vi "SwissSPAD Live_Write HDF5 Header.vi"(8 "error in (no error)":errorcluster, 9 "Gate Names":string[](array[string]), 10 "Current Data Set":i32, 11 "ref in":T1 format="%.0x") -> (0 "Error Out":errorcluster, 1 "Notebook Message":string, 2 "# Image Sets":u32, 3 "ref out":T1 format="%.0x", 5 "# Datasets in Series":i32)   [LabVIEW 2021]
uses:
  <vilib>/addons/h5labview2/base/hid_t.ctl
  SwissSPAD Live_HDF5 Header Sections.ctl
  SwissSPAD Live_File Information.ctl
  SwissSPAD Live_Settings List.ctl
  SwissSPAD Live_SSx PCB Version.ctl
  SwissSPAD Live_Image ROI Information.ctl
  Phasor/Image Binning Options.ctl
  <vilib>/addons/h5labview2/base/lib_path.vi
  <vilib>/addons/h5labview2/base/H5Equery.vi
  <vilib>/addons/h5labview2/dataset/H5Dwrite.llb/H5Dwrite.xnode
  <vilib>/addons/h5labview2/group/H5G.lvlib
  Variant/Variant to Data/Variant to Data.lvlib
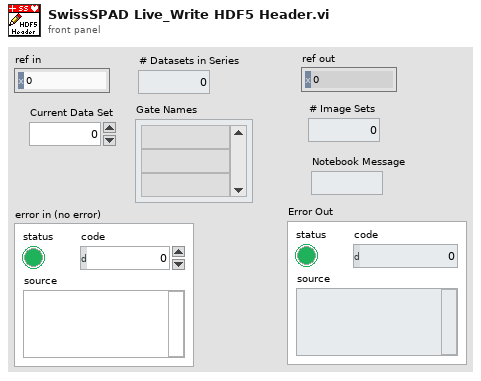
[diagram p1: front panel]
types:
  T1 = typedef "hid_t.ctl" = i32
  T2 = typedef "SwissSPAD Live_HDF5 Header Sections.ctl" = enum16{"File Information", "SwissSPAD Detector Information", "DAQ Parameters", "Image Information", "Metadata"}
  T3 = typedef "SwissSPAD Live_Settings List.ctl" = enum16{"FPGA:Bottom Half", "FPGA:Top Half", "FPGA:Bottom Bitfile Path", "FPGA:Top Bitfile Path", "FPGA:Bottom Bitstream Version", "FPGA:Top Bitstream Version", "FPGA:Auto Reset FPGA", "FPGA:Bottom FPGA Serial Number", "FPGA:Top FPGA Serial Number", "FPGA:Detector PCB Version", "Acquisition Parameters:Microlens", "Acquisition Parameters:SS2 DAQ Parameters", "Acquisition Parameters:Gate Configuration Array", "Acquisition Parameters:SS3 DAQ Parameters", "Acquisition Parameters:Buffer Size (# 8-bit Gates)", "File Information:File Information", "File Information:# Datasets in Series", "File Information:Scrambled File Flag", "File Information:SS3 Gate Slip Correction", "File Information:SS3 Hot Pixel Mismatch Detection", "File Information:Delay between Datasets", "File Information:Save Sum of All Gates Preview", "Image Parameters:Image ROI Information", "Image Parameters:Image Binning Options", "Image Parameters:SS3 Displayed Image", "Image Parameters:Image Display Options", "Image Parameters:Use Histogram Cursors", "Image Parameter:FPGA Data to Display", "UI Settings:Histogram Bins Number", "UI Settings:Use Image Display Options", "UI Settings:Verbose Settings", "UI Settings:Verbose Saving"}
  T4 = typedef "SwissSPAD Live_File Information.ctl" = cluster{"File Folder":path, "File Name":string, "File Index":u32, "Author":string, "Sample":string, "Compression":bool, "Compression Level":u8}
  T5 = typedef "SwissSPAD Live_SSx PCB Version.ctl" = enum16{"unknown", "SS2 PCB1", "SS2 PCB2", "SS3 PCB1"}
  T6 = typedef "Image Binning Options.ctl" = cluster{"Use Image Binning":bool, "X Bin":i32, "Y Bin":i32}
  T7 = typedef "SwissSPAD Live_Image ROI Information.ctl" = cluster{"Save ROI Only":bool, "Left":u16, "Top":u16, "Right":u16, "Bottom":u16, "Use Current ROI":bool}
  T8 = typedef "Fluorescence Lifetime Parameters v3.ctl" = cluster{"# Pixel X":i32, "# Pixel Y":i32, "# Gates":i32, "# Datasets":i32, "Gate Image Exposure":dbl[unit], "Macrotime Gate Separation":dbl[unit], "Nanotime Gate Separation":dbl[unit], "Gate Width":dbl[unit], "Laser Period":dbl[unit], "SYNC Period":dbl[unit], "Gate Image Integration":dbl[unit]}
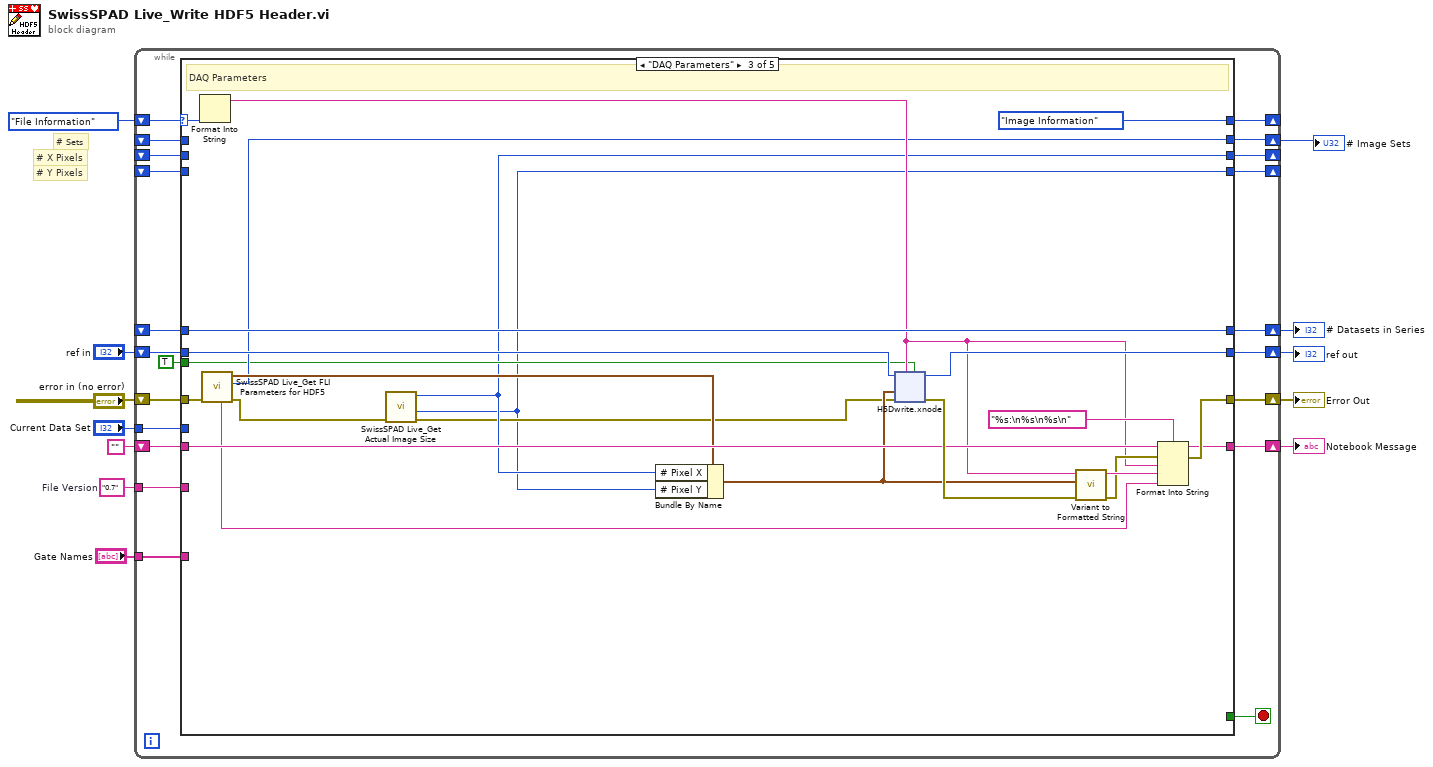
[diagram p0: block diagram]
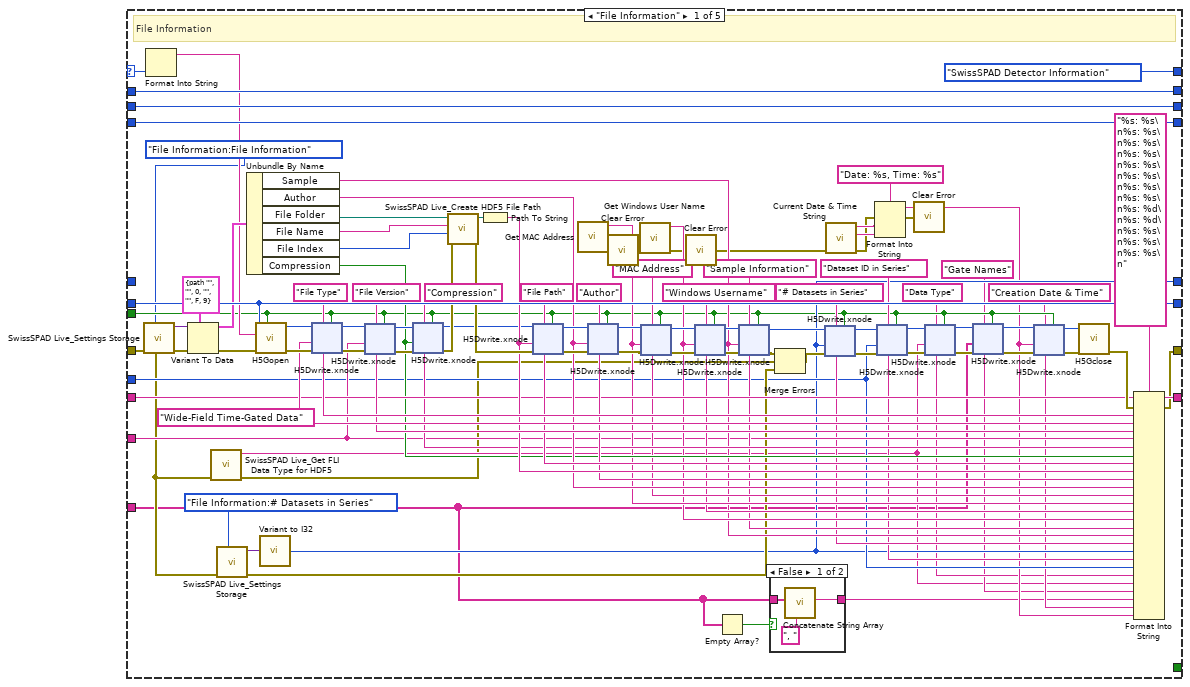
[diagram p2: hidden frame]
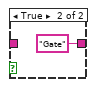
[diagram p3: hidden frame]
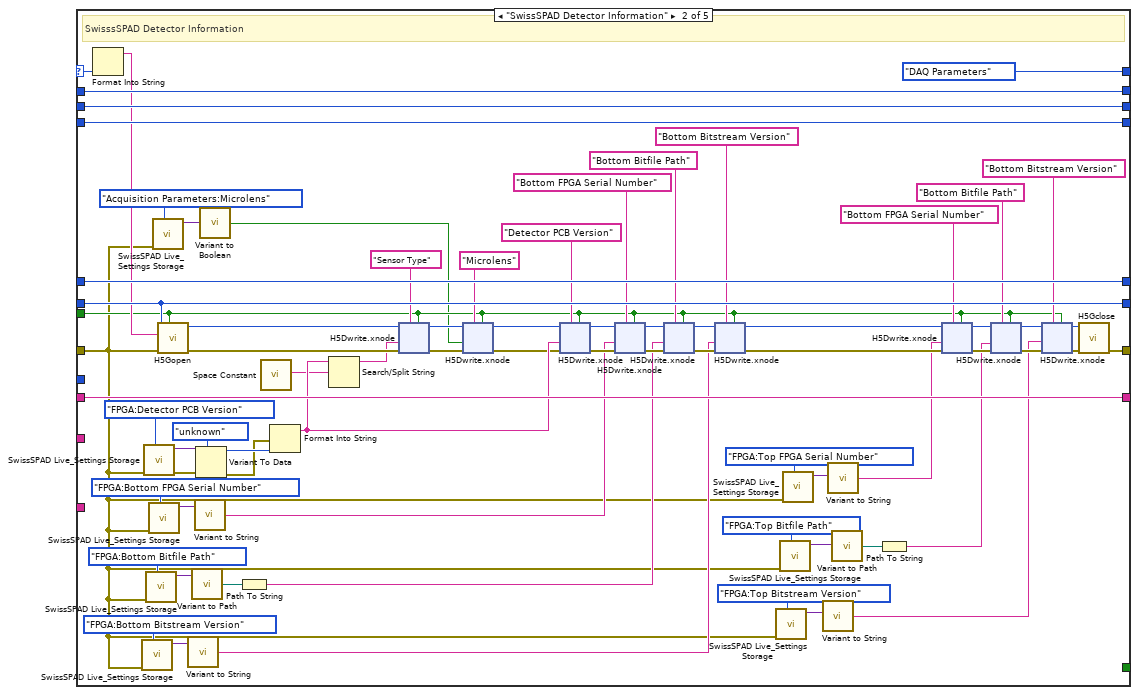
[diagram p4: hidden frame]
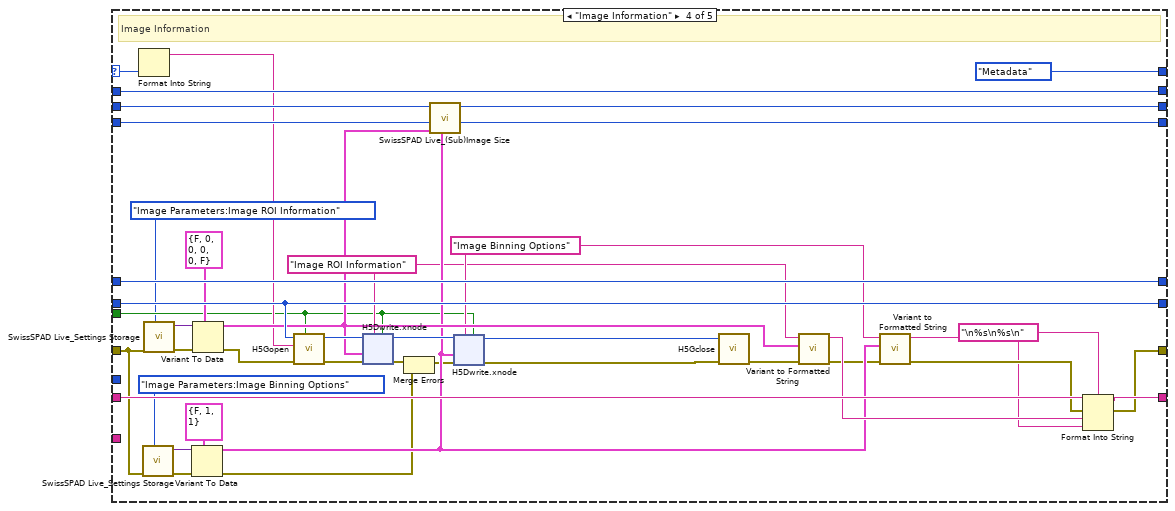
[diagram p5: hidden frame]
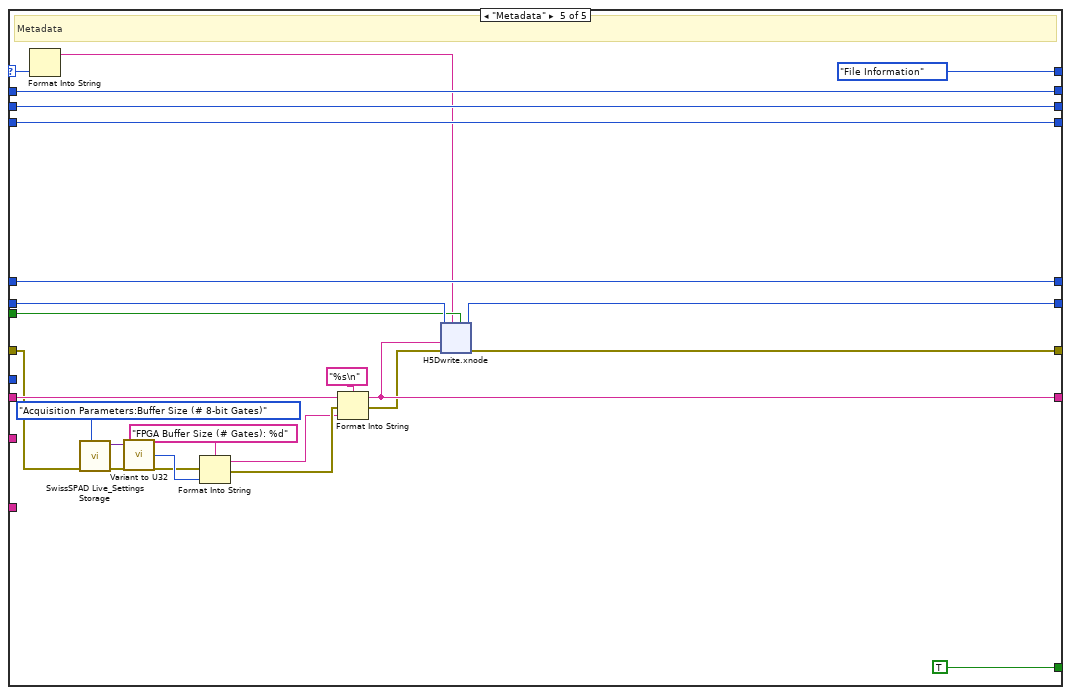
[diagram p6: hidden frame]
diagram:
  w3 = "0.7"  # File Version
  # "# Y Pixels"
  # "# X Pixels"
  # "# Sets"
  n1 = while {
    shift-right: [w30] -> w10
    shift-left: "ref in" -> [w32]
    shift-right: [w31] -> w9
    shift-left: "error in (no error)" -> [w33]
    shift-right: [w27] -> w6
    shift-left: _ -> [w26]
    tunnel: "Current Data Set" -> [w25]
    shift-right: [w24] -> w7
    shift-left: _ -> [w23]
    shift-right: [w28] -> w4
    shift-left: "" -> [w22]
    shift-right: [w20] -> _
    shift-left: _ -> [w21]
    shift-right: [w18] -> _
    shift-left: _ -> [w19]
    tunnel: w3 -> [w17]
    shift-right: [w15] -> _
    shift-left: SwissSPAD_Live_HDF5_Header_Sections."File Information" -> [w16]
    tunnel: "Gate Names" -> [w13]
    stop <- w14 stop-if-true
    n2 = case shown="\"DAQ Parameters\"" w16 {
      selector: w16 -> [w72 w445 w630 w679 w750]
      tunnel: w33 -> [w54 w383 w645 w687 w756]
      tunnel: w32 -> [w122 w446 w639 w705 w768]
      tunnel: [w96 w442 w641 w697 w759] -> w31
      tunnel: [w122 w446 w644 w705 w767] -> w30
      tunnel: TRUE ("replace? (F)") -> [w47 w384 w627 w672 w766]
      tunnel: [w99 w441 w638 w698 w761] -> w28
      tunnel: [w55 w451 w636 w701 w764] -> w27
      tunnel: w26 -> [_ w451 w636 w701 w764]
      tunnel: w25 -> [w61 _ _ _ _]
      tunnel: [w95 w450 w628 w702 w763] -> w24
      tunnel: w23 -> [w95 w450 _ w702 w763]
      tunnel: w22 -> [w94 w441 w637 w699 w762]
      tunnel: [w93 w449 w626 w693 w758] -> w20
      tunnel: w21 -> [w93 w449 _ w694 w758]
      tunnel: [w92 w448 w623 w691 w757] -> w18
      tunnel: w19 -> [w92 w448 _ w692 w757]
      tunnel: w17 -> [w73 _ _ _ _]
      tunnel: [SwissSPAD_Live_HDF5_Header_Sections."SwissSPAD Detector Information" SwissSPAD_Live_HDF5_Header_Sections."DAQ Parameters" SwissSPAD_Live_HDF5_Header_Sections."Image Information" SwissSPAD_Live_HDF5_Header_Sections."Metadata" SwissSPAD_Live_HDF5_Header_Sections."File Information"] -> w15
      tunnel: [_ _ _ _ TRUE] -> w14
      tunnel: w13 -> [w39 _ _ _ _]
      frame "File Information" {
        w43 = "Gate Names" ("dataset name")
        w44 = "Data Type" ("dataset name")
        w62 = "Dataset ID in Series" ("name")
        w63 = "# Datasets in Series" ("name")
        w77 = "Windows Username" ("dataset name")
        w79 = "MAC Address" ("dataset name")
        w87 = "Compression" ("dataset name")
        w45 = "Creation Date & Time" ("dataset name")
        w75 = "Sample Information" ("dataset name")
        w101 = "Author" ("dataset name")
        w103 = "File Path" ("dataset name")
        w105 = "Wide-Field Time-Gated Data" ("dataset name")
        w106 = "File Type" ("dataset name")
        w104 = "File Version" ("dataset name")
        # "File Information"
        n3 = call "SwissSPAD Live_Settings Storage.vi"("Settings List"=SwissSPAD_Live_Settings_List."File Information:File Information", "Error In"=w54) -> ("Error Out"=w128:errorcluster, "Variant Data out"=w36:variant)  [unwired: 8 in]
        n4 = Format Into String(w72) -> (resulting string=w71:string)  [unwired: 3 in, 1 out]
        n5 = Variant To Data(error in=w128, type=T4 {"File Folder"=path "", "File Name"="", "File Index"=0, "Author"="", "Sample"="", "Compression"=FALSE, "Compression Level"=9} ("File Information"), Variant=w36) -> (data=w120:T4, error out=w121:errorcluster)
        n6 = call "SwissSPAD Live_Get FLI Data Type for HDF5.vi"("error in (no error)"=w54) -> ("error out"=w41:errorcluster, "Data Type"=w42:string)  [unwired: 9 in]
        n7 = call "SwissSPAD Live_Settings Storage.vi"("Settings List"=SwissSPAD_Live_Settings_List."File Information:# Datasets in Series", "Error In"=w54) -> ("Error Out"=w64:errorcluster, "Variant Data out"=w34:variant)  [unwired: 8 in]
        n8 = Unbundle By Name(w120) -> ("Sample"=w74:string, "Author"=w100:string, "File Folder"=w119:path, "File Name"=w118:string, "File Index"=w117:u32, "Compression"=w86:bool)
        n9 = call <vilib>:"H5Gopen.vi"("create? (F)"=w47, "error in (no error)"=w121, "name"=w71, "ref in"=w122) -> ("error out"=w125:errorcluster, "group out"=w126:T1)  [unwired: 6 in]
        n10 = call "Variant to I32.vi"("Variant"=w34) -> ("Value"=w55:i32)  [unwired: 8 in]
        n11 = xnode "H5Dwrite.xnode"("replace? (F)"=w47, "dataset name"=w106, "error in (no error)"=w125, "data"=w105, "ref in"=w126) -> ("error out"=w124:errorcluster, "ref out"=w123:i32)  [unwired: 2 in, 1 out]
        n12 = xnode "H5Dwrite.xnode"("replace? (F)"=w47, "dataset name"=w104, "error in (no error)"=w124, "data"=w73, "ref in"=w123) -> ("error out"=w91:errorcluster, "ref out"=w89:i32)  [unwired: 2 in, 1 out]
        n13 = xnode "H5Dwrite.xnode"("replace? (F)"=w47, "dataset name"=w87, "error in (no error)"=w91, "data"=w86, "ref in"=w89) -> ("error out"=w90:errorcluster, "ref out"=w88:i32)  [unwired: 2 in, 1 out]
        n14 = call "SwissSPAD Live_Create HDF5 File Path.vi"("error in (no error)"=w90, "File Index"=w117, "File Name"=w118, "File Folder"=w119) -> ("error out"=w116:errorcluster, "File path"=w115:path)  [unwired: 6 in]
        n15 = Path To String(path=w115) -> (string=w102:string)
        n16 = xnode "H5Dwrite.xnode"("replace? (F)"=w47, "dataset name"=w103, "error in (no error)"=w116, "data"=w102, "ref in"=w88) -> ("error out"=w113:errorcluster, "ref out"=w114:i32)  [unwired: 2 in, 1 out]
        n17 = call "Get MAC Address.vi"() -> ("Error Out"=w60:errorcluster, "MAC address"=w78:string)  [unwired: 10 in]
        n18 = xnode "H5Dwrite.xnode"("replace? (F)"=w47, "dataset name"=w101, "error in (no error)"=w113, "data"=w100, "ref in"=w114) -> ("error out"=w85:errorcluster, "ref out"=w84:i32)  [unwired: 2 in, 1 out]
        n19 = call "Clear Error.vi"("Error In"=w60) -> ("no Error Out"=w59:errorcluster)  [unwired: 8 in]
        n20 = call "Get Windows User Name.vi"("Error In"=w59) -> ("Error Out"=w58:errorcluster, "User Name"=w76:string)  [unwired: 9 in]
        n21 = xnode "H5Dwrite.xnode"("replace? (F)"=w47, "dataset name"=w79, "error in (no error)"=w85, "data"=w78, "ref in"=w84) -> ("error out"=w83:errorcluster, "ref out"=w82:i32)  [unwired: 2 in, 1 out]
        n22 = call "Clear Error.vi"("Error In"=w58) -> ("no Error Out"=w57:errorcluster)  [unwired: 8 in]
        n23 = xnode "H5Dwrite.xnode"("replace? (F)"=w47, "dataset name"=w77, "error in (no error)"=w83, "data"=w76, "ref in"=w82) -> ("error out"=w80:errorcluster, "ref out"=w81:i32)  [unwired: 2 in, 1 out]
        n24 = Empty Array?(array=w39) -> (empty?=w38:bool)
        n25 = xnode "H5Dwrite.xnode"("replace? (F)"=w47, "dataset name"=w75, "error in (no error)"=w80, "data"=w74, "ref in"=w81) -> ("error out"=w67:errorcluster, "ref out"=w66:i32)  [unwired: 2 in, 1 out]
        n26 = case shown="False" w38 {
          tunnel: [w130 "Gate" ("Formatted String")] -> w40
          tunnel: w39 -> [w129 _]
          frame False {
            n27 = call "Concatenate String Array.vi"("Separator (TAB)"=", ", "String Array"=w129) -> ("Formatted String"=w130:string)  [unwired: 9 in]
          }
          frame True {
          }
        }
        n28 = Merge Errors(w67, w41, w64) -> (w65:errorcluster)
        n29 = xnode "H5Dwrite.xnode"("replace? (F)"=w47, "dataset name"=w63, "error in (no error)"=w65, "data"=w55, "ref in"=w66) -> ("error out"=w69:errorcluster, "ref out"=w68:i32)  [unwired: 2 in, 1 out]
        n30 = call "Current Date & Time String.vi"("Error In"=w57) -> ("Error Out"=w109:errorcluster, "time string"=w110:string, "date string"=w111:string)  [unwired: 8 in]
        n31 = Format Into String(format string="Date: %s, Time: %s", error in=w109, w111, w110) -> (resulting string=w46:string, error out=w56:errorcluster)  [unwired: 1 in]
        n32 = xnode "H5Dwrite.xnode"("replace? (F)"=w47, "dataset name"=w62, "error in (no error)"=w69, "data"=w61, "ref in"=w68) -> ("error out"=w52:errorcluster, "ref out"=w53:T1)  [unwired: 2 in, 1 out]
        n33 = call "Clear Error.vi"("Error In"=w56) -> ()  [unwired: 8 in, 1 out]
        n34 = xnode "H5Dwrite.xnode"("replace? (F)"=w47, "dataset name"=w44, "error in (no error)"=w52, "data"=w42, "ref in"=w53) -> ("error out"=w51:errorcluster, "ref out"=w50:T1)  [unwired: 2 in, 1 out]
        n35 = xnode "H5Dwrite.xnode"("replace? (F)"=w47, "dataset name"=w43, "error in (no error)"=w51, "data"=w39, "ref in"=w50) -> ("error out"=w48:errorcluster, "ref out"=w49:T1)  [unwired: 2 in, 1 out]
        n36 = xnode "H5Dwrite.xnode"("replace? (F)"=w47, "dataset name"=w45, "error in (no error)"=w48, "data"=w46, "ref in"=w49) -> ("error out"=w98:errorcluster, "ref out"=w112:i32)  [unwired: 2 in, 1 out]
        n37 = call <vilib>:"H5Gclose.vi"("error in (no error)"=w98, "group in"=w112) -> ("error out"=w97:errorcluster)  [unwired: 9 in]
        n38 = Format Into String(format string="%s: %s\n%s: %s\n%s: %s\n%s: %s\n%s: %s\n%s: %s\n%s: %s\n%s: %s\n%s: %d\n%s: %d\n%s: %s\n%s: %s\n%s: %s\n", initial string=w94, error in=w97, w106, w105, w104, w73, w87, w86, w103, w102, w101, w100, w79, w78, w77, w76, w75, w74, w63, w55, w62, w61, w44, w42, w43, w40, w45, w46) -> (resulting string=w99:string, error out=w96:errorcluster)
      }
      frame "SwissSPAD Detector Information" {
        # "SwisssSPAD Detector Information"
        n39 = Format Into String(w445) -> (resulting string=w444:string)  [unwired: 3 in, 1 out]
        n40 = call "SwissSPAD Live_Settings Storage.vi"("Settings List"=SwissSPAD_Live_Settings_List."FPGA:Bottom Bitstream Version", "Error In"=w383) -> ("Variant Data out"=w412:variant)  [unwired: 8 in, 1 out]
        n41 = call "SwissSPAD Live_Settings Storage.vi"("Settings List"=SwissSPAD_Live_Settings_List."FPGA:Detector PCB Version", "Error In"=w383) -> ("Error Out"=w439:errorcluster, "Variant Data out"=w409:variant)  [unwired: 8 in]
        n42 = call "SwissSPAD Live_Settings Storage.vi"("Settings List"=SwissSPAD_Live_Settings_List."FPGA:Bottom Bitfile Path", "Error In"=w383) -> ("Variant Data out"=w411:variant)  [unwired: 8 in, 1 out]
        n43 = call "SwissSPAD Live_Settings Storage.vi"("Settings List"=SwissSPAD_Live_Settings_List."FPGA:Bottom FPGA Serial Number", "Error In"=w383) -> ("Variant Data out"=w410:variant)  [unwired: 8 in, 1 out]
        n44 = call "SwissSPAD Live_Settings Storage.vi"("Settings List"=SwissSPAD_Live_Settings_List."Acquisition Parameters:Microlens", "Error In"=w383) -> ("Variant Data out"=w382:variant)  [unwired: 8 in, 1 out]
        n45 = call <vilib>:"H5Gopen.vi"("create? (F)"=w384, "error in (no error)"=w383, "name"=w444, "ref in"=w446) -> ("error out"=w443:errorcluster, "group out"=w447:T1)  [unwired: 6 in]
        n46 = call "Variant to String.vi"("Variant"=w412) -> ("String"=w418:string)  [unwired: 8 in]
        n47 = call "Variant to Path.vi"("Variant"=w411) -> ("Path"=w420:path)  [unwired: 8 in]
        n48 = call "Variant to String.vi"("Variant"=w410) -> ("String"=w421:string)  [unwired: 8 in]
        n49 = Variant To Data(error in=w439, type=SwissSPAD_Live_SSx_PCB_Version."unknown" ("Detector PCB Version"), Variant=w409) -> (data=w437:T5, error out=w436:errorcluster)
        n50 = call "Variant to Boolean.vi"("Variant"=w382) -> ("Value"=w380:bool)  [unwired: 8 in]
        n51 = Path To String(path=w420) -> (string=w419:string)
        n52 = call <vilib>:"Space Constant.vi"() -> ("String"=w433:string)
        n53 = Format Into String(error in=w436, w437) -> (resulting string=w434:string)  [unwired: 2 in, 1 out]
        n54 = Search/Split String(string=w434, search string/char (-)=w433) -> (substring before match=w432:string)  [unwired: 1 in, 2 out]
        n55 = xnode "H5Dwrite.xnode"("replace? (F)"=w384, "dataset name"="Sensor Type", "error in (no error)"=w443, "data"=w432, "ref in"=w447) -> ("error out"=w389:errorcluster, "ref out"=w387:i32)  [unwired: 2 in, 1 out]
        n56 = xnode "H5Dwrite.xnode"("replace? (F)"=w384, "dataset name"="Microlens", "error in (no error)"=w389, "data"=w380, "ref in"=w387) -> ("error out"=w388:errorcluster, "ref out"=w386:i32)  [unwired: 2 in, 1 out]
        n57 = xnode "H5Dwrite.xnode"("replace? (F)"=w384, "dataset name"="Detector PCB Version", "error in (no error)"=w388, "data"=w434, "ref in"=w386) -> ("error out"=w431:errorcluster, "ref out"=w430:i32)  [unwired: 2 in, 1 out]
        n58 = xnode "H5Dwrite.xnode"("replace? (F)"=w384, "dataset name"="Bottom FPGA Serial Number", "error in (no error)"=w431, "data"=w421, "ref in"=w430) -> ("error out"=w428:errorcluster, "ref out"=w427:i32)  [unwired: 2 in, 1 out]
        n59 = xnode "H5Dwrite.xnode"("replace? (F)"=w384, "dataset name"="Bottom Bitfile Path", "error in (no error)"=w428, "data"=w419, "ref in"=w427) -> ("error out"=w425:errorcluster, "ref out"=w423:i32)  [unwired: 2 in, 1 out]
        n60 = xnode "H5Dwrite.xnode"("replace? (F)"=w384, "dataset name"="Bottom Bitstream Version", "error in (no error)"=w425, "data"=w418, "ref in"=w423) -> ("error out"=w424:errorcluster, "ref out"=w391:i32)  [unwired: 2 in, 1 out]
        n61 = call "SwissSPAD Live_Settings Storage.vi"("Settings List"=SwissSPAD_Live_Settings_List."FPGA:Top Bitstream Version", "Error In"=w383) -> ("Variant Data out"=w406:variant)  [unwired: 8 in, 1 out]
        n62 = call "SwissSPAD Live_Settings Storage.vi"("Settings List"=SwissSPAD_Live_Settings_List."FPGA:Top Bitfile Path", "Error In"=w383) -> ("Variant Data out"=w407:variant)  [unwired: 8 in, 1 out]
        n63 = call "SwissSPAD Live_Settings Storage.vi"("Settings List"=SwissSPAD_Live_Settings_List."FPGA:Top FPGA Serial Number", "Error In"=w383) -> ("Variant Data out"=w408:variant)  [unwired: 8 in, 1 out]
        n64 = call "Variant to String.vi"("Variant"=w406) -> ("String"=w392:string)  [unwired: 8 in]
        n65 = call "Variant to String.vi"("Variant"=w408) -> ("String"=w394:string)  [unwired: 8 in]
        n66 = call "Variant to Path.vi"("Variant"=w407) -> ("Path"=w402:path)  [unwired: 8 in]
        n67 = Path To String(path=w402) -> (string=w393:string)
        n68 = xnode "H5Dwrite.xnode"("replace? (F)"=w384, "dataset name"="Bottom FPGA Serial Number", "data"=w394, "ref in"=w391) -> ("error out"=w400:errorcluster, "ref out"=w399:i32)  [unwired: 3 in, 1 out]
        n69 = xnode "H5Dwrite.xnode"("replace? (F)"=w384, "dataset name"="Bottom Bitfile Path", "error in (no error)"=w400, "data"=w393, "ref in"=w399) -> ("error out"=w397:errorcluster, "ref out"=w396:T1)  [unwired: 2 in, 1 out]
        n70 = xnode "H5Dwrite.xnode"("replace? (F)"=w384, "dataset name"="Bottom Bitstream Version", "error in (no error)"=w397, "data"=w392, "ref in"=w396) -> ("ref out"=w390:T1)  [unwired: 2 in, 2 out]
        n71 = call <vilib>:"H5Gclose.vi"("error in (no error)"=w424, "group in"=w390) -> ("error out"=w442:errorcluster)  [unwired: 9 in]
      }
      frame "DAQ Parameters" {
        # "DAQ Parameters"
        n72 = Format Into String(w630) -> (resulting string=w629:string)  [unwired: 3 in, 1 out]
        n73 = call "SwissSPAD Live_Get FLI Parameters for HDF5.vi"("error in (no error)"=w645) -> ("error out"=w625:errorcluster, "# Sets"=w628:u32, "Acquisition Parameters"=w635:T8, "Metadata String"=w634:string)  [unwired: 7 in]
        n74 = call "SwissSPAD Live_Get Actual Image Size.vi"("error in (no error)"=w625) -> ("error out"=w624:errorcluster, "Y size"=w623:i32, "X size"=w626:i32)  [unwired: 8 in]
        n75 = Bundle By Name(cluster=w635, "# Pixel X"=w626, "# Pixel Y"=w623) -> (w633:T8)
        n76 = xnode "H5Dwrite.xnode"("replace? (F)"=w627, "dataset name"=w629, "error in (no error)"=w624, "data"=w633, "ref in"=w639) -> ("error out"=w642:errorcluster, "ref out"=w644:i32)  [unwired: 2 in, 1 out]
        n77 = call "Variant to Formatted String.vi"("Error In"=w642, "Variant"=w633, "Label"=w629) -> ("Error Out"=w631:errorcluster, "String"=w643:string)  [unwired: 7 in]
        n78 = Format Into String(format string="%s:\n%s\n%s\n", initial string=w637, error in=w631, w629, w643, w634) -> (resulting string=w638:string, error out=w641:errorcluster)
      }
      frame "Image Information" {
        w682 = "Image Binning Options" ("name")
        w673 = "Image ROI Information" ("name")
        # "Image Information"
        n79 = Format Into String(w679) -> (resulting string=w678:string)  [unwired: 3 in, 1 out]
        n80 = call "SwissSPAD Live_Settings Storage.vi"("Settings List"=SwissSPAD_Live_Settings_List."Image Parameters:Image Binning Options", "Error In"=w687) -> ("Error Out"=w686:errorcluster, "Variant Data out"=w668:variant)  [unwired: 8 in]
        n81 = call "SwissSPAD Live_Settings Storage.vi"("Settings List"=SwissSPAD_Live_Settings_List."Image Parameters:Image ROI Information", "Error In"=w687) -> ("Error Out"=w706:errorcluster, "Variant Data out"=w665:variant)  [unwired: 8 in]
        n82 = Variant To Data(error in=w686, type=T6 {"Use Image Binning"=FALSE, "X Bin"=1, "Y Bin"=1} ("Image Binning Options"), Variant=w668) -> (data=w683:T6, error out=w675:errorcluster)
        n83 = Variant To Data(error in=w706, type=T7 {"Save ROI Only"=FALSE, "Left"=0, "Top"=0, "Right"=0, "Bottom"=0, "Use Current ROI"=FALSE} ("Image Information"), Variant=w665) -> (data=w690:T7, error out=w677:errorcluster)
        n84 = call <vilib>:"H5Gopen.vi"("create? (F)"=w672, "error in (no error)"=w677, "name"=w678, "ref in"=w705) -> ("error out"=w703:errorcluster, "group out"=w704:T1)  [unwired: 6 in]
        n85 = xnode "H5Dwrite.xnode"("replace? (F)"=w672, "dataset name"=w673, "error in (no error)"=w703, "data"=w690, "ref in"=w704) -> ("error out"=w689:errorcluster, "ref out"=w688:i32)  [unwired: 2 in, 1 out]
        n86 = Merge Errors(w689, w675) -> (w676:errorcluster)
        n87 = call "SwissSPAD Live_(Sub)Image Size.vi"("Image Binning Options"=w683, "Image Information"=w690, "# Pixel Y in"=w692, "# Pixel X in"=w694) -> ("# Pixel Y out"=w691:i32, "# Pixel X out"=w693:i32)  [unwired: 6 in]
        n88 = xnode "H5Dwrite.xnode"("replace? (F)"=w672, "dataset name"=w682, "error in (no error)"=w676, "data"=w683, "ref in"=w688) -> ("error out"=w669:errorcluster, "ref out"=w670:i32)  [unwired: 2 in, 1 out]
        n89 = call <vilib>:"H5Gclose.vi"("error in (no error)"=w669, "group in"=w670) -> ("error out"=w684:errorcluster)  [unwired: 9 in]
        n90 = call "Variant to Formatted String.vi"("Error In"=w684, "Variant"=w690, "Label"=w673) -> ("Error Out"=w674:errorcluster, "String"=w696:string)  [unwired: 7 in]
        n91 = call "Variant to Formatted String.vi"("Error In"=w674, "Variant"=w683, "Label"=w682) -> ("Error Out"=w681:errorcluster, "String"=w680:string)  [unwired: 7 in]
        n92 = Format Into String(format string="\n%s\n%s\n", initial string=w699, error in=w681, w696, w680) -> (resulting string=w698:string, error out=w697:errorcluster)
      }
      frame "Metadata" {
        # "Metadata"
        n93 = Format Into String(w750) -> (resulting string=w749:string)  [unwired: 3 in, 1 out]
        n94 = call "SwissSPAD Live_Settings Storage.vi"("Settings List"=SwissSPAD_Live_Settings_List."Acquisition Parameters:Buffer Size (# 8-bit Gates)", "Error In"=w756) -> ("Error Out"=w754:errorcluster, "Variant Data out"=w746:variant)  [unwired: 8 in]
        n95 = call "Variant to U32.vi"("Variant"=w746) -> ("Value"=w755:u32)  [unwired: 8 in]
        n96 = Format Into String(format string="FPGA Buffer Size (# Gates): %d", error in=w754, w755) -> (resulting string=w751:string, error out=w753:errorcluster)  [unwired: 1 in]
        n97 = Format Into String(format string="%s\n", initial string=w762, error in=w753, w751) -> (resulting string=w761:string, error out=w760:errorcluster)
        n98 = xnode "H5Dwrite.xnode"("replace? (F)"=w766, "dataset name"=w749, "error in (no error)"=w760, "data"=w761, "ref in"=w768) -> ("error out"=w759:errorcluster, "ref out"=w767:i32)  [unwired: 2 in, 1 out]
      }
    }
  }
  "ref out" <- w10
  "Error Out" <- w9
  "Notebook Message" <- w4
  "# Image Sets" <- w7
  "# Datasets in Series" <- w6
